vi "System Check.vi"(8 "Error In":errorcluster, 11 "Target Configuration VI Path":path) -> (0 "Error Out":errorcluster, 2 "Current LV Version":string, 3 "Saved LV Version":string)   [LabVIEW 2014, in "LMH-LINX.lvlib"]
uses:
  <vilib>/MakerHub/LINX/LMH-LINX.lvlib
  <vilib>/MakerHub/Toolbox/LMH-Toolbox.lvlib
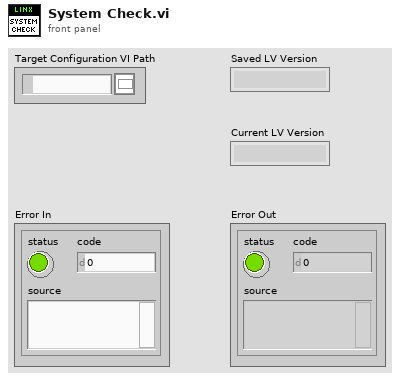
[diagram p1: front panel]
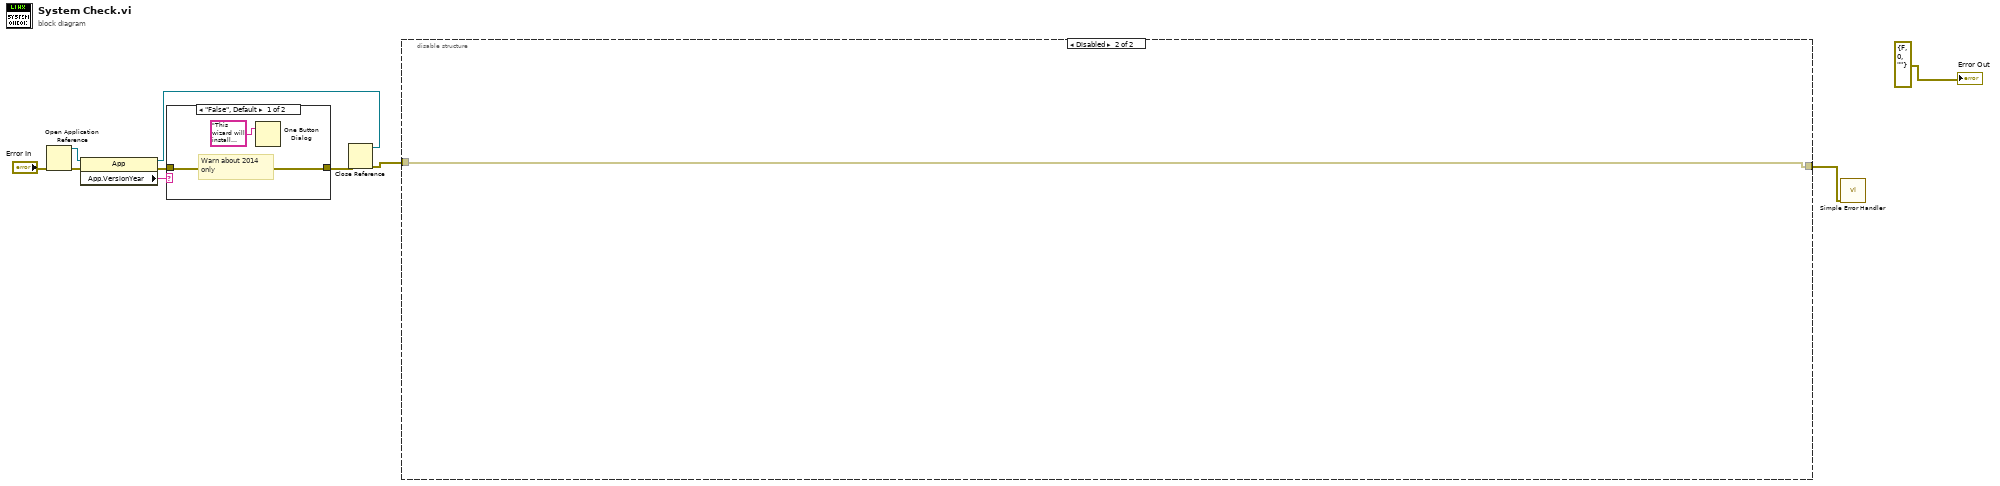
[diagram p0: block diagram]
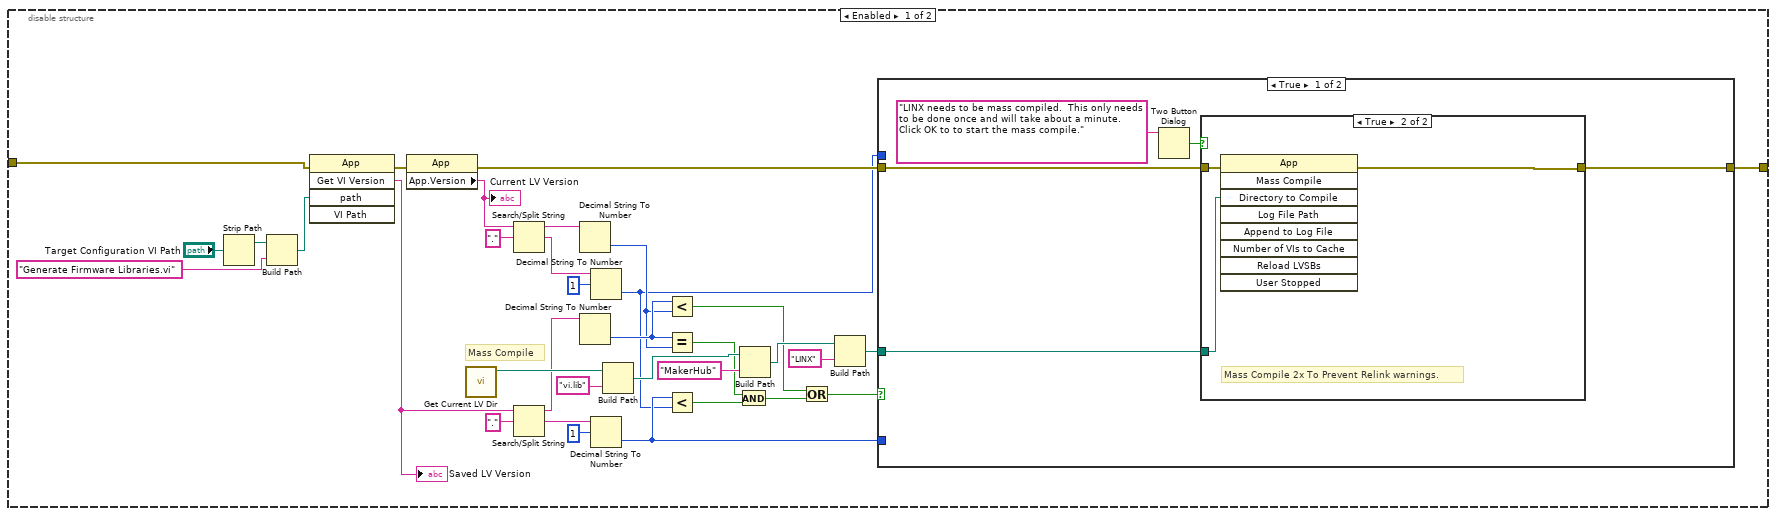
[diagram p2: hidden frame]
diagram:
  n1 = Open Application Reference(8:"Error In") -> (0:w6:errorcluster, 3:w8:refnum<vi>)  [unwired: 3 in]
  n2 = property class="App"(reference=w8, error in=w6) -> (reference out=w7:refnum<vi>, error out=w3:errorcluster, "App.VersionYear"=w5:string)
  n3 = case shown="\"False\", Default" w5 {
    tunnel: [w12 w13] -> w4
    tunnel: w3 -> [w12 w13]
    frame "False", Default {
      # "Warn about 2014\nonly"
      n4 = One Button Dialog(message="This wizard will install LabVIEW 2014 support to the target device.  \nYou will only be able to connect to and use the device from LabVIEW 2014.") -> ()  [unwired: 1 in, 1 out]
    }
    frame "2014" {
    }
  }
  n5 = Close Reference(reference=w7, error in (no error)=w4) -> (error out=w10:errorcluster)
  n6 = disable-structure shown="Disabled" {
    disable-tunnel: w10 -> [w40 w58]
    disable-tunnel: [w15 w58] -> w2
    frame Enabled {
      # "Mass Compile"
      n7 = Strip Path(path="Target Configuration VI Path") -> (stripped path=w25:path)  [unwired: 1 out]
      n8 = Build Path(base path=w25, name or relative path="Generate Firmware Libraries.vi") -> (appended path=w27:path)
      n9 = invoke class="App" method="Get VI Version"(error in=w40, "path"=w27) -> (error out=w39:errorcluster, "GetVIVers"=w37:string)  [unwired: 3 in, 3 out]
      "Saved LV Version" <- w37
      n10 = property class="App"(error in=w39) -> (error out=w38:errorcluster, "App.Version"=w31:string)  [unwired: 1 in, 1 out]
      "Current LV Version" <- w31
      n11 = call <vilib>:"Get Current LV Dir.vi"() -> ("This LV Directory"=w46:path)  [unwired: 10 in, 1 out]
      n12 = Search/Split String(string=w31, search string/char (-)=".") -> (substring before match=w32:string, match + rest of string=w29:string)  [unwired: 1 in, 1 out]
      n13 = Search/Split String(string=w37, search string/char (-)=".") -> (substring before match=w33:string, match + rest of string=w35:string)  [unwired: 1 in, 1 out]
      n14 = Decimal String To Number(string=w32) -> (number=w23:i32)  [unwired: 2 in, 1 out]
      n15 = Decimal String To Number(string=w33) -> (number=w24:i32)  [unwired: 2 in, 1 out]
      n16 = Decimal String To Number(string=w29, offset=1) -> (number=w19:i32)  [unwired: 1 in, 1 out]
      n17 = Decimal String To Number(string=w35, offset=1) -> (number=w20:i32)  [unwired: 1 in, 1 out]
      n18 = Build Path(base path=w46, name or relative path="vi.lib") -> (appended path=w42:path)
      n19 = Less?(x=w24, y=w23) -> (x < y?=w18:bool)
      n20 = Equal?(x=w24, y=w23) -> (x = y?=w22:bool)
      n21 = Less?(x=w20, y=w19) -> (x < y?=w21:bool)
      n22 = And(x=w22, y=w21) -> (x .and. y?=w17:bool)
      n23 = Build Path(base path=w42, name or relative path="MakerHub") -> (appended path=w41:path)
      n24 = Or(x=w18, y=w17) -> (x .or. y?=w16:bool)
      n25 = Build Path(base path=w41, name or relative path="LINX") -> (appended path=w47:path)
      n26 = case shown="True" w16 {
        tunnel: w20 -> [_ _]
        tunnel: w19 -> [_ _]
        tunnel: [w50 w57] -> w15
        tunnel: w38 -> [w49 w57]
        tunnel: w47 -> [w48 _]
        frame True {
          n27 = Two Button Dialog(message="LINX needs to be mass compiled.  This only needs to be done once and will take about a minute.  Click OK to to start the mass compile.") -> (T button?=w51:bool)  [unwired: 2 in]
          n28 = case shown="True" w51 {
            tunnel: [w53 w54] -> w50
            tunnel: w49 -> [w53 w56]
            tunnel: w48 -> [_ w55]
            frame False {
              # "Cancel Mass Compile"
            }
            frame True {
              # "Mass Compile 2x To Prevent Relink warnings."
              n29 = invoke class="App" method="Mass Compile"(error in=w56, "Directory to Compile"=w55) -> (error out=w54:errorcluster)  [unwired: 7 in, 8 out]
            }
          }
        }
        frame False {
          # "Saved Version Is Not Older Than This Version"
        }
      }
    }
    frame Disabled {
    }
  }
  n30 = call <vilib>:"Simple Error Handler.vi"("error in (no error)"=w2) -> ()  [unwired: 4 in, 5 out]
  "Error Out" <- errorcluster {"status"=FALSE, "code"=0, "source"=""} ("error constant")
